vi "Complex IIR Filter (real signal).vi"(2 "init/cont (init:F)":bool, 3 "Forward Coefficients":cdb[](array[numeric]), 4 "Reverse Coefficients":cdb[](array[numeric]), 5 "X":dbl[](array[numeric])) -> (0 "error":i32, 1 "Filtered X":cdb[](array[numeric]))   [LabVIEW 2010, in "NI_AALBase.lvlib"]
uses:
  NI_AALBase.lvlib
  lvanlys.dll
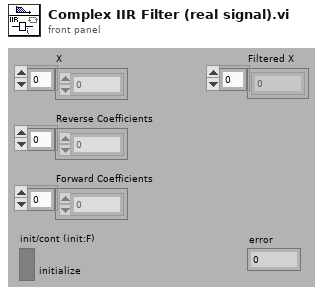
[diagram p1: front panel]
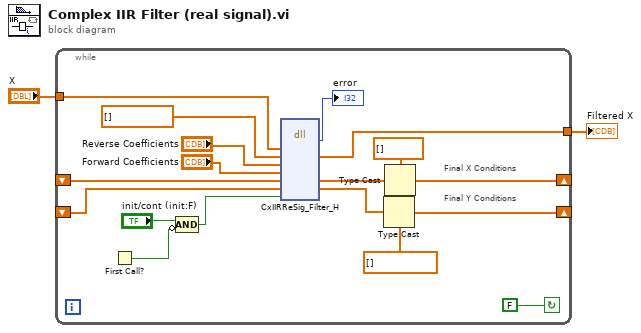
[diagram p0: block diagram]
diagram:
  n1 = while {
    shift-left: _ -> [w12]
    shift-right: [w19] -> _
    shift-left: _ -> [w10]
    shift-right: [w20] -> _
    tunnel: "X" -> [w15]
    tunnel: [w6] -> w1
    stop <- FALSE continue-if-true
    # "Final Y Conditions"
    # "Final X Conditions"
    n2 = First Call?() -> (First Call?: T/F=w14:bool)
    n3 = Compound Arithmetic op=AND("init/cont (init:F)", invert w14) -> (w13:bool)
    n4 = dll-call lib="C:/Program Files/National Instruments/LabVIEW 2010/resource/lvanlys.*" fn="CxIIRReSig_Filter_H"("xH"=w15, "Y"=cdb[] [], "Reverse Coefficients"="Reverse Coefficients", "Forward Coefficients"="Forward Coefficients", "x1H"=w10, "type for the shift register"=w12, w13) -> (→"error":i32, "Y"=w6:cdb[], "x1H"=w9:dbl[], "type for the shift register"=w11:cdb[])  [unwired: 7 in, 2 out]
    n5 = Type Cast(type=cdb[] [] ("type for the shift register"), x=w11) -> (*(type *) &x=w19:cdb[])
    n6 = Type Cast(type=dbl[] [], x=w9) -> (*(type *) &x=w20:dbl[])
  }
  "Filtered X" <- w1
